vi "1-16.vi"() -> ()   [LabVIEW 2022 SP3]
panel:
  out "循环次数":dbl
  out "随机数":dbl
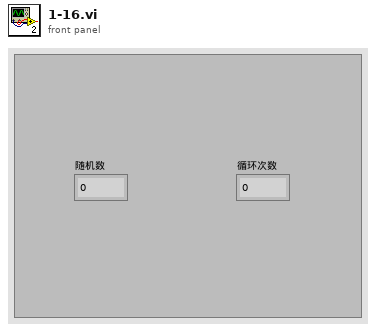
[diagram p1: front panel]
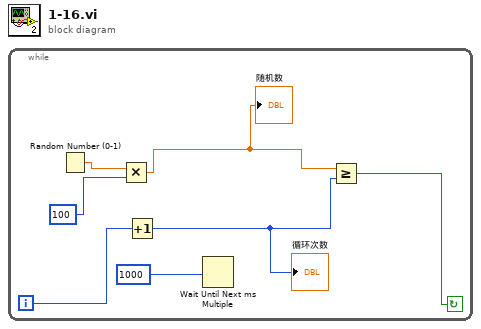
[diagram p0: block diagram]
diagram:
  n1 = while {
    i -> [w4]
    stop <- w3 continue-if-true
    n2 = Random Number (0-1)() -> (number: 0 to 1=w7:dbl)
    n3 = Multiply(x=w7, y=100) -> (x*y=w5:dbl)
    "随机数" <- w5
    n4 = Increment(x=w4) -> (x+1=w2:i32)
    "循环次数" <- w2
    n5 = Wait Until Next ms Multiple(millisecond multiple=1000) -> ()  [unwired: 1 out]
    n6 = Greater Or Equal?(x=w5, y=w2) -> (x >= y?=w3:bool)
  }
